vi "组合框.vi"() -> ()   [LabVIEW 2018]
panel:
  in  "停止":bool
  out "密码显示":string
  out "正常显示":string
  in  "组合框":string(combo)
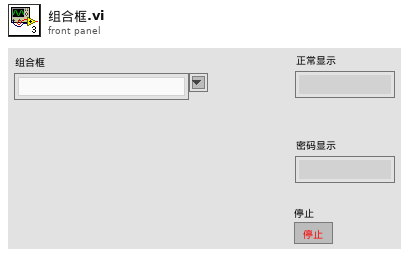
[diagram p1: front panel]
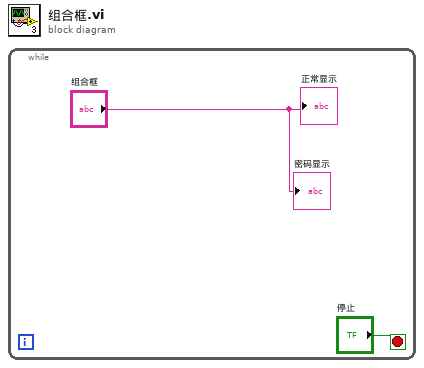
[diagram p0: block diagram]
diagram:
  n1 = while {
    stop <- "停止" stop-if-true
    "正常显示" <- "组合框"
    "密码显示" <- "组合框"
  }
